vi "SSL Detection Frame Simple Estimator.vi"(5 "dt":dbl, 7 "Enable":bool=TRUE, 10 "Field Size":T1, 11 "Detection Frame In":T2 {"robots_blue"."height" format="%+4.3f"; "robots_blue"."pixel_y" format="%+4.3f"; "robots_blue"."pixel_x" format="%+4.3f"; "robots_blue"."orientation" format="%+4.3f"; "robots_blue"."y" format="%+4.3f"; "robots_blue"."confidence" format="%4.3f"; "robots_blue"."x" format="%+4.3f"; "robots_yellow"."height" format="%+4.3f"; "robots_yellow"."pixel_y" format="%+4.3f"; "robots_yellow"."pixel_x" format="%+4.3f"; "robots_yellow"."orientation" format="%+4.3f"; "robots_yellow"."y" format="%+4.3f"; "robots_yellow"."confidence" format="%4.3f"; "robots_yellow"."x" format="%+4.3f"}) -> (2 "Field Size Out":T1, 3 "Detection Frame Out":T2 {"robots_blue"."height" format="%+4.3f"; "robots_blue"."pixel_y" format="%+4.3f"; "robots_blue"."pixel_x" format="%+4.3f"; "robots_blue"."orientation" format="%+4.3f"; "robots_blue"."y" format="%+4.3f"; "robots_blue"."confidence" format="%4.3f"; "robots_blue"."x" format="%+4.3f"; "robots_yellow"."height" format="%+4.3f"; "robots_yellow"."pixel_y" format="%+4.3f"; "robots_yellow"."pixel_x" format="%+4.3f"; "robots_yellow"."orientation" format="%+4.3f"; "robots_yellow"."y" format="%+4.3f"; "robots_yellow"."confidence" format="%4.3f"; "robots_yellow"."x" format="%+4.3f"})   [LabVIEW 2018]
uses:
  SSL Detection Frame.ctl
  SSL Detection Robot.ctl
  <vilib>/Analysis/Matrix/Datatypes/RealMatrix.ctl
  SSL Detection Ball.ctl
  <vilib>/Analysis/Matrix/NI_Matrix.lvlib
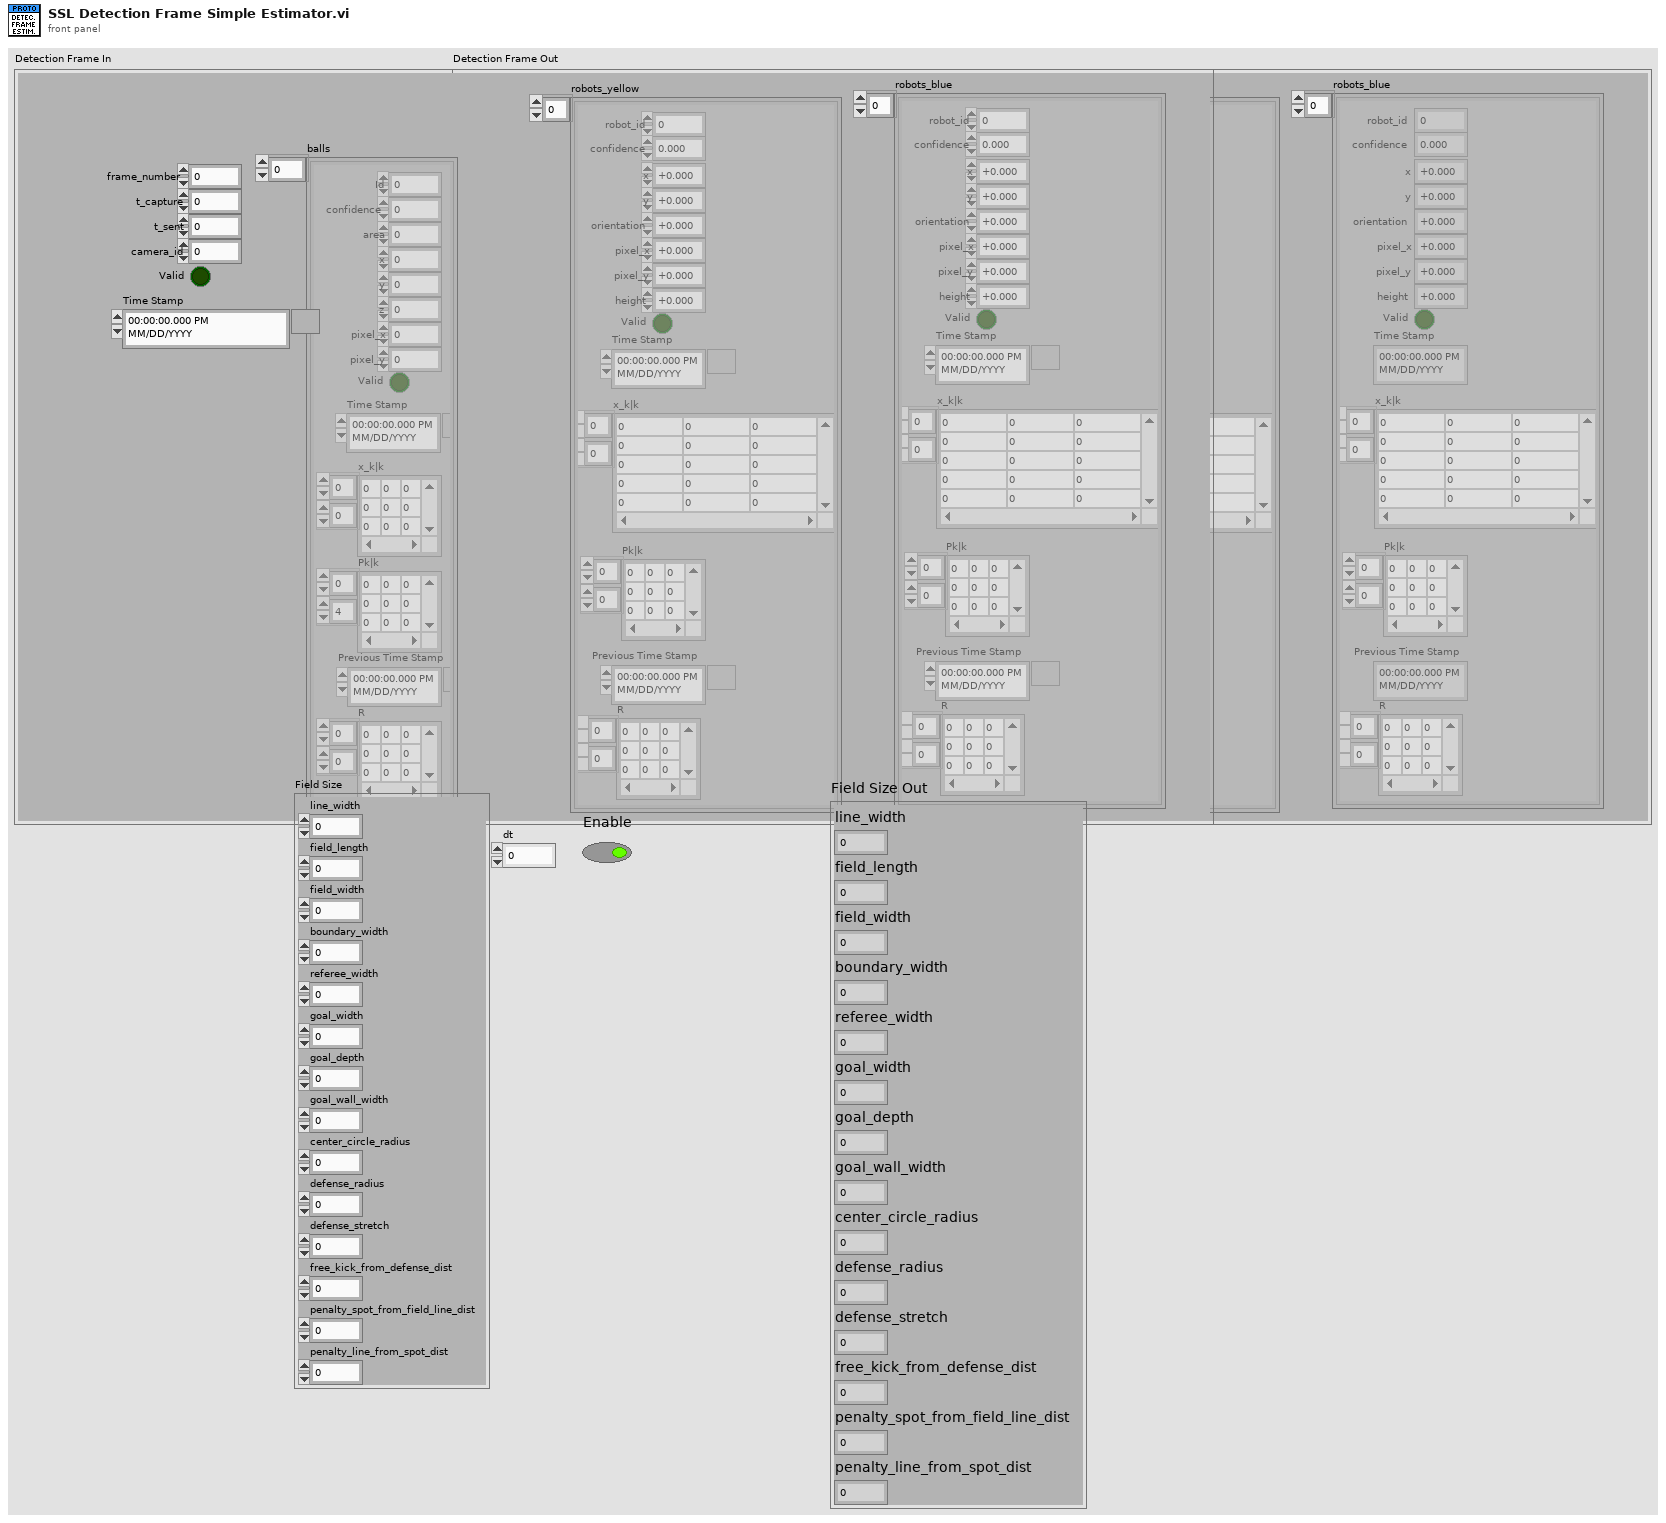
[diagram p1: front panel]
types:
  T1 = cluster{"line_width":u32, "field_length":u32, "field_width":u32, "boundary_width":u32, "referee_width":u32, "goal_width":u32, "goal_depth":u32, "goal_wall_width":u32, "center_circle_radius":u32, "defense_radius":u32, "defense_stretch":u32, "free_kick_from_defense_dist":u32, "penalty_spot_from_field_line_dist":u32, "penalty_line_from_spot_dist":u32}
  T2 = typedef "SSL Detection Frame.ctl" = cluster{"frame_number":u32, "t_capture":dbl, "t_sent":dbl, "camera_id":u32, "robots_yellow":T3[], "robots_blue":T3[], "balls":T5[], "Valid":bool, "Time Stamp":timestamp}
  T3 = typedef "SSL Detection Robot.ctl" = cluster{"x":sgl, "robot_id":u32, "confidence":sgl, "y":sgl, "orientation":sgl, "pixel_x":sgl, "pixel_y":sgl, "height":sgl, "Valid":bool, "Time Stamp":timestamp, "x_k|k":T4, "Pk|k":T4, "Previous Time Stamp":timestamp, "R":T4}
  T4 = typedef "NI_Matrix.lvlib/RealMatrix.ctl" = dbl[][]
  T5 = typedef "SSL Detection Ball.ctl" = cluster{"x":sgl, "area":u32, "confidence":sgl, "y":sgl, "z":sgl, "pixel_x":sgl, "pixel_y":sgl, "Valid":bool, "Time Stamp":timestamp, "x_k|k":T4, "Pk|k":T4, "Id":u32, "Previous Time Stamp":timestamp, "R":T4}
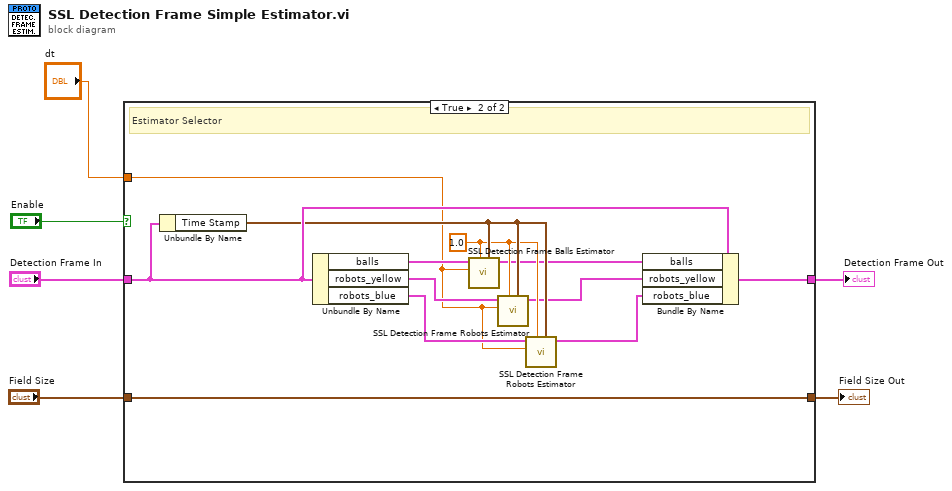
[diagram p0: block diagram]
diagram:
  n1 = case shown="True" "Enable" {
    tunnel: [w8 w20] -> w6
    tunnel: "Detection Frame In" -> [w8 w18]
    tunnel: "Field Size" -> [w7 w19]
    tunnel: [w7 w19] -> w3
    tunnel: "dt" -> [_ w9]
    frame False {
    }
    frame True {
      w13 = 1.0 ("Life Time")
      # "Estimator Selector"
      n2 = Unbundle By Name(w18) -> ("Time Stamp"=w17:timestamp)
      n3 = Unbundle By Name(w18) -> ("balls"=w15:T5[], "robots_yellow"=w16:T3[], "robots_blue"=w14:T3[])
      n4 = call "SSL Detection Frame Balls Estimator.vi"("Time Stamp"=w17, "Life Time"=w13, "dt"=w9, "Balls"=w15) -> ("Est balls"=w10:T5[])  [unwired: 7 in]
      n5 = call "SSL Detection Frame Robots Estimator.vi"("Time Stamp"=w17, "Life Time"=w13, "dt"=w9, "Robots"=w16) -> ("Est. Robots"=w12:T3[])  [unwired: 7 in]
      n6 = call "SSL Detection Frame Robots Estimator.vi"("Time Stamp"=w17, "Life Time"=w13, "dt"=w9, "Robots"=w14) -> ("Est. Robots"=w11:T3[])  [unwired: 7 in]
      n7 = Bundle By Name(cluster=w18, "balls"=w10, "robots_yellow"=w12, "robots_blue"=w11) -> (w20:T2)
    }
  }
  "Detection Frame Out" <- w6
  "Field Size Out" <- w3
